vi "Get Group Delay - Halfband Decimators.vi"(10 "sampling rate in":dbl, 11 "# of hb decimators":i32) -> (0 "group delay (s)":dbl, 2 "sampling rate out":dbl)   [LabVIEW 2021, in "Digitizer Control.lvclass"]
doc: "Returns the group delay of the halfband decimators in the acquistion path."
uses:
  Digitizer Control.lvclass
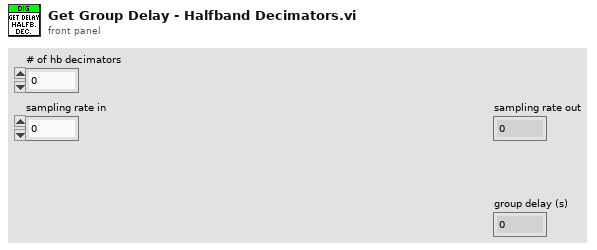
[diagram p1: front panel]
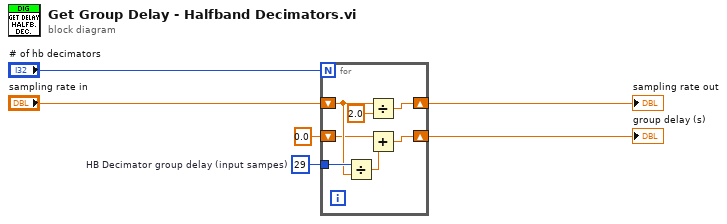
[diagram p0: block diagram]
diagram:
  w1 = 29  # HB Decimator group delay (input sampes)
  n1 = for {
    N: "# of hb decimators" -> [_]
    tunnel: w1 -> [w13]
    shift-right: [w10] -> w5
    shift-left: "sampling rate in" -> [w12]
    shift-right: [w8] -> w3
    shift-left: 0.0 -> [w9]
    n2 = Divide(x=w13, y=w12) -> (x/y=w7:dbl)
    n3 = Divide(x=w12, y=2.0) -> (x/y=w10:dbl)
    n4 = Add(x=w9, y=w7) -> (x+y=w8:dbl)
  }
  "sampling rate out" <- w5
  "group delay (s)" <- w3
